vi "JAPCtestsubscribeINT.vi"(8 "error in (no error)":errorcluster, 11 "URL":string="VAC.VGHA_41677/PR") -> (0 "error out":errorcluster, 2 "JAPCint":string, 3 "Numeric":i16)   [LabVIEW 2014]
uses:
  <userlib>/_RADE/RIO/JAPC/classes/JSubscribe/openJAPCSubscribe.vi
  <userlib>/_RADE/RIO/JAPC/classes/JSubscribe/JAPCSubscribe.vi
  <userlib>/_RADE/RIO/JAPC/classes/JSubscribe/JSubscribe.lvclass
panel:
  out "Data":variant
  out "Loop":i32
  in  "stop":bool
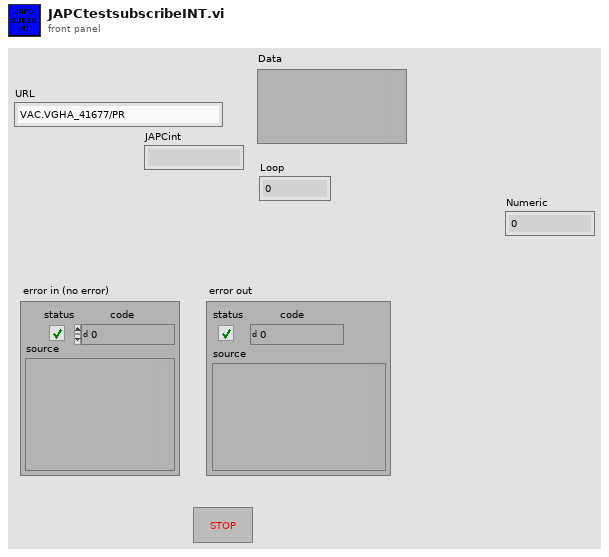
[diagram p1: front panel]
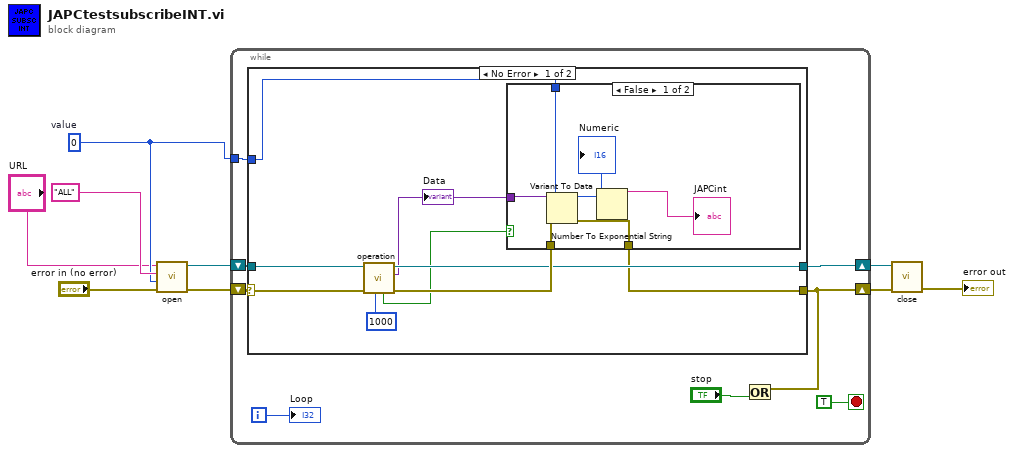
[diagram p0: block diagram]
diagram:
  w2 = i16 0  # value
  n1 = call-poly <userlib>:"open.vi"("error in (no error)"="error in (no error)", "Data type"=w2, "Cycle"="ALL", "URL"="URL") -> ("error out"=w7:errorcluster, "Object out"=w6:refnum<class "JSubscribe.lvclass">)  [unwired: 6 in]
  n2 = while {
    shift-right: [w14] -> w5
    shift-left: w7 -> [w17]
    shift-right: [w12] -> w4
    shift-left: w6 -> [w13]
    tunnel: w2 -> [w11]
    i -> [w15]
    stop <- TRUE stop-if-true
    n3 = case shown="No Error" w17 {
      selector: w17 -> [w18 w35]
      tunnel: [w24 w35] -> w14
      tunnel: w13 -> [w19 w34]
      tunnel: [w25 w34] -> w12
      tunnel: w11 -> [w23 _]
      frame No Error {
        n4 = call-poly <userlib>:"operation.vi"("Timeout (10000 ms)"=1000, "error in (no error)"=w18, "Object in"=w19) -> ("error out"=w26:errorcluster, "Data"=w22:variant, "Object out"=w25:refnum<class "JSubscribe.lvclass">, "Timeout?"=w20:bool)  [unwired: 3 in, 2 out]
        "Data" <- w22
        n5 = case shown="False" w20 {
          tunnel: w26 -> [w32 w33]
          tunnel: [w29 w33] -> w24
          tunnel: w22 -> [w31 _]
          tunnel: w23 -> [w30 _]
          frame False {
            n6 = Variant To Data(error in=w32, type=w30, Variant=w31) -> (data=w28:i16, error out=w29:errorcluster)
            "Numeric" <- w28
            n7 = Number To Exponential String(number=w28) -> (E-format string=→"JAPCint":string)  [unwired: 3 in]
          }
          frame True {
          }
        }
      }
      frame Error {
      }
    }
    n8 = Or(x=w14, y="stop") -> ()  [unwired: 1 out]
    "Loop" <- w15
  }
  n9 = call-dynamic "close.vi"("error in (no error)"=w5, "Object in"=w4) -> ("error out"=→"error out":errorcluster)  [unwired: 9 in]
